vi "Konvolucio MCAN120803 Example_0004 Write.vi"   [LabVIEW 2011]
uses:
  <instrlib>/Konvolucio MCAN120803/Types/MessageType.ctl
  <instrlib>/Konvolucio MCAN120803/Public/Attributes/AttrSetTermination.vi
  <instrlib>/Konvolucio MCAN120803/Konvolucio MCAN120803.lvlib
types:
  T1 = typedef "Konvolucio MCAN120803.lvlib/MessageType.ctl" = cluster{"TimeStamp":timestamp, "ArbitrationId":u32, "IsRemote":u8, "DataLength":u8, "Data":u8[]}
  T2 = typedef "Konvolucio MCAN120803.lvlib/CanHandleType.ctl" = cluster{"AdapterDevice":refnum<k24>}
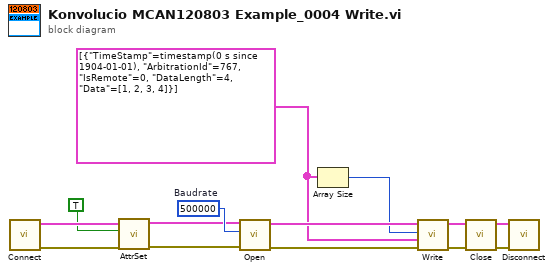
[diagram p0: block diagram]
diagram:
  w11 = T1[] [{"TimeStamp"=timestamp(0 s since 1904-01-01), "ArbitrationId"=767, "IsRemote"=0, "DataLength"=4, "Data"=[1, 2, 3, 4]}] ("Messages")
  w14 = u32 500000  # Baudrate
  n1 = call <instrlib>:"Connect.vi"() -> ("error out"=w9:errorcluster, "CanHandleOut"=w7:T2)  [unwired: 10 in]
  n2 = call-poly <instrlib>:"AttrSet.vi"("error in"=w9, "Enabled"=TRUE, "CanHandleIn"=w7) -> ("error out"=w8:errorcluster, "CanHandleOut"=w6:T2)  [unwired: 6 in]
  n3 = call <instrlib>:"Open.vi"("error in"=w8, "Baudrate"=w14, "CanHandleIn"=w6) -> ("error out"=w13:errorcluster, "CanHandleOut"=w12:T2)  [unwired: 7 in]
  n4 = Array Size(array=w11) -> (size(s)=w10:i32)
  n5 = call <instrlib>:"Write.vi"("error in"=w13, "Messages"=w11, "Number to Write"=w10, "CanHandleIn"=w12) -> ("error out"=w4:errorcluster, "CanHandleOut"=w3:T2)  [unwired: 4 in]
  n6 = call <instrlib>:"Close.vi"("error in"=w4, "CanHandleIn"=w3) -> ("error out"=w2:errorcluster, "CanHandleOut"=w1:T2)  [unwired: 8 in]
  n7 = call <instrlib>:"Disconnect.vi"("error in"=w2, "CanHandleIn"=w1) -> ()  [unwired: 9 in, 1 out]
